vi "Add Oneof Index To Metadata.vi"(11 "message metadata":T1) -> (3 "message metadata with oneof index":T1)   [LabVIEW 2019, in "gRPC Template Creation Utility.lvlib"]
uses:
  gRPC Template Creation Utility.lvlib
  TypeDefs/Message Metadata (Scripting).ctl
  TypeDefs/Message Element Metadata (Scripting).ctl
  TypeDefs/Message Element Type.ctl
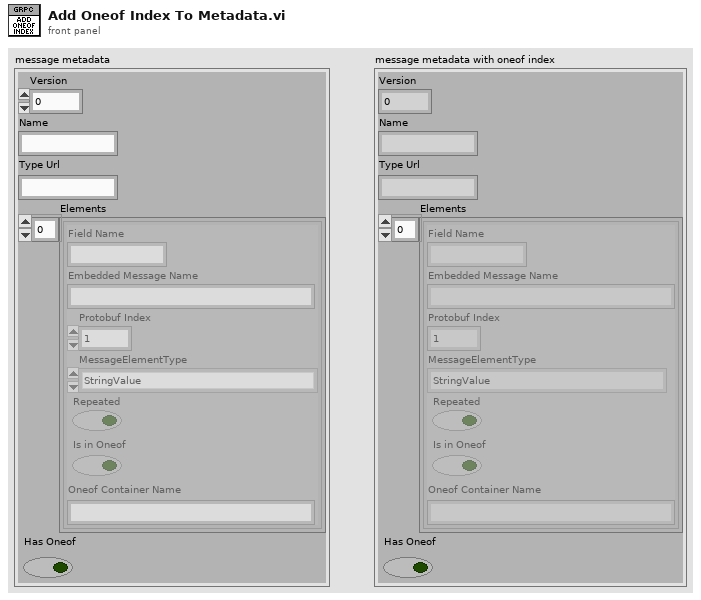
[diagram p1: front panel]
types:
  T1 = typedef "gRPC Template Creation Utility.lvlib/Message Metadata (Scripting).ctl" = cluster{"Version":i32, "Name":string, "Type Url":string, "Elements":T2[], "Has Oneof":bool}
  T2 = typedef "gRPC Template Creation Utility.lvlib/Message Element Metadata (Scripting).ctl" = cluster{"Field Name":string, "Embedded Message Name":string, "Protobuf Index":i32, "MessageElementType":T3, "Repeated":bool, "Is in Oneof":bool, "Oneof Container Name":string}
  T3 = typedef "gRPC Template Creation Utility.lvlib/Message Element Type.ctl" = enum32{"Int32Value", "FloatValue", "DoubleValue", "BoolValue", "StringValue", "MessageValue", "Int64Value", "UInt32Value", "UInt64Value", "EnumValue", "Bytes", "Fixed64", "Fixed32", "SFixed64", "SFixed32", "SInt64", "SInt32"}
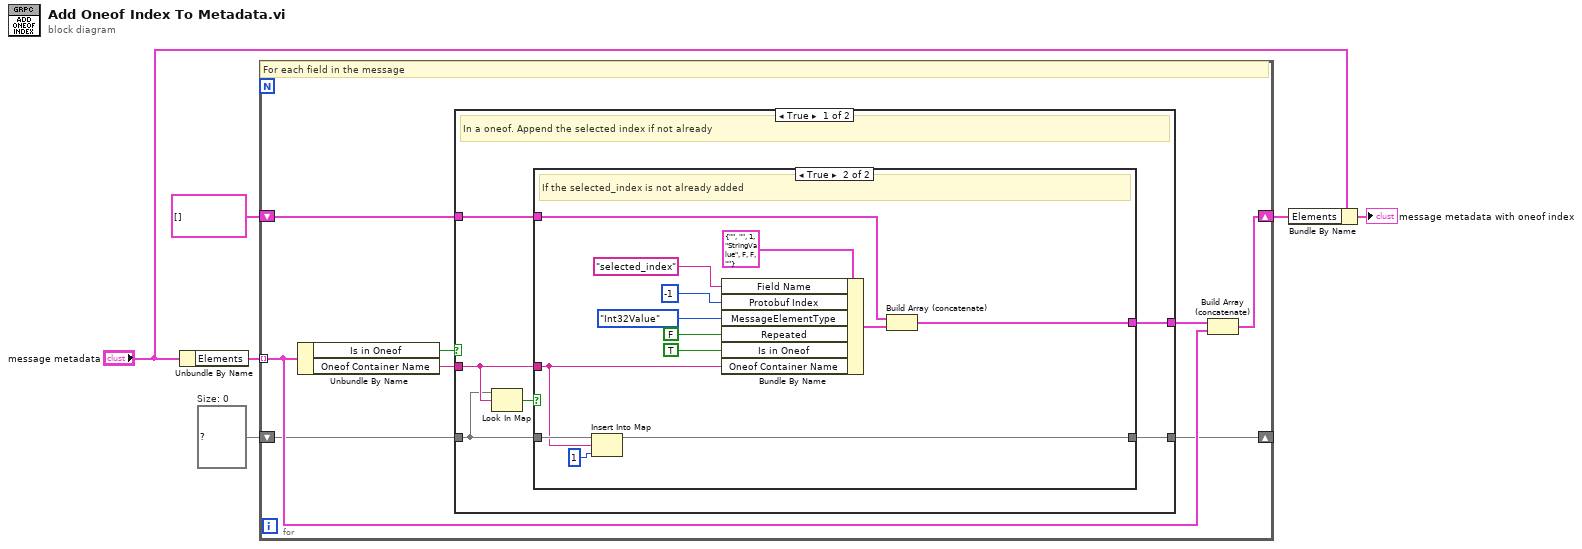
[diagram p0: block diagram]
diagram:
  w5 = map{string, i32} {}  # Size: 0
  n1 = Unbundle By Name("message metadata") -> ("Elements"=w6:T2[])
  n2 = for {
    shift-right: [w9] -> w3
    shift-left: T2[] [] -> [w13]
    tunnel: w6 -> [w10] mode=indexing
    shift-right: [w7] -> _
    shift-left: w5 -> [w8]
    # "For each field in the message"
    n3 = Unbundle By Name(w10) -> ("Is in Oneof"=w14:bool, "Oneof Container Name"=w12:string)
    n4 = case shown="True" w14 {
      tunnel: w13 -> [w20 w37]
      tunnel: w12 -> [w18 _]
      tunnel: [w19 w37] -> w11
      tunnel: w8 -> [w16 w36]
      tunnel: [w15 w36] -> w7
      frame True {
        # "In a oneof. Append the selected index if not already"
        n5 = Look In Map(map=w16, key=w18) -> (key not found?=w17:bool)  [unwired: 1 in, 1 out]
        n6 = case shown="True" w17 {
          tunnel: w18 -> [_ w26]
          tunnel: w20 -> [w22 w29]
          tunnel: [w22 w28] -> w19
          tunnel: w16 -> [w21 w27]
          tunnel: [w21 w24] -> w15
          frame False {
          }
          frame True {
            # "If the selected_index is not already added"
            n7 = Insert Into Map(map in=w27, key=w26, value=1) -> (map out=w24:map{string, i32})  [unwired: 2 out]
            n8 = Bundle By Name(cluster=T2 {"Field Name"="", "Embedded Message Name"="", "Protobuf Index"=1, "MessageElementType"=enum."StringValue", "Repeated"=FALSE, "Is in Oneof"=FALSE, "Oneof Container Name"=""} ("MessageElementMetadata"), "Field Name"="selected_index", "Protobuf Index"=-1, "MessageElementType"=Message_Element_Type."Int32Value", "Repeated"=FALSE, "Is in Oneof"=TRUE, "Oneof Container Name"=w26) -> (w30:T2)
            n9 = Build Array (concatenate)(w29, w30) -> (w28:T2[])
          }
        }
      }
      frame False {
        # "Not in a oneof. Just append to the metadata fields"
      }
    }
    n10 = Build Array (concatenate)(w11, w10) -> (w9:T2[])
  }
  n11 = Bundle By Name(cluster="message metadata", "Elements"=w3) -> (→"message metadata with oneof index":T1)
